vi "Find_Screen_Res.vi"(8 "error in (no error)":errorcluster, 10 "Front Panel.WinBounds":T1) -> (0 "error out":errorcluster, 2 "Width & Height":cluster{"Width":i32, "Height":i32})   [LabVIEW 2018]
uses:
  <vilib>/Utility/miscctls.llb/LVRectTypeDef.ctl
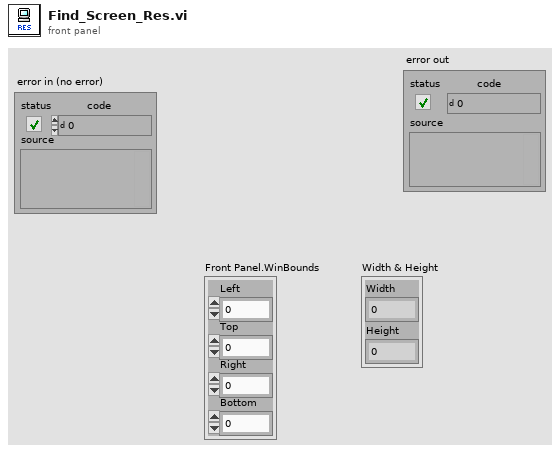
[diagram p1: front panel]
types:
  T1 = typedef "LVRectTypeDef.ctl" = cluster{"Left":i16, "Top":i16, "Right":i16, "Bottom":i16}
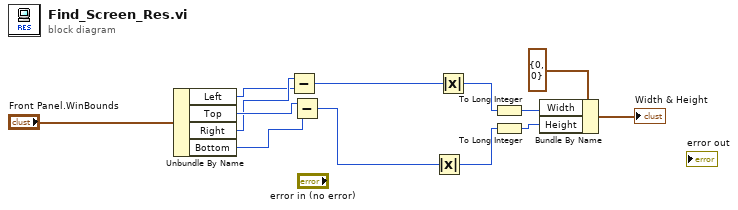
[diagram p0: block diagram]
diagram:
  n1 = Unbundle By Name("Front Panel.WinBounds") -> ("Left"=w9:i16, "Top"=w12:i16, "Right"=w10:i16, "Bottom"=w11:i16)
  n2 = Subtract(x=w10, y=w9) -> (x-y=w7:i16)
  n3 = Subtract(x=w12, y=w11) -> (x-y=w8:i16)
  n4 = Absolute Value(x=w8) -> (abs(x)=w2:i16)
  n5 = Absolute Value(x=w7) -> (abs(x)=w4:i16)
  n6 = To Long Integer(number=w4) -> (32bit integer=w3:i32)
  n7 = To Long Integer(number=w2) -> (32bit integer=w1:i32)
  n8 = Bundle By Name(cluster=cluster{"Width":i32, "Height":i32} {"Width"=0, "Height"=0} ("Width & Height"), "Width"=w3, "Height"=w1) -> (→"Width & Height":cluster{"Width":i32, "Height":i32})
